vi "FTW-CodeGen-Initialize.vi"(5 "XRef":refnum<vi>) -> (4 "State Out":T1)   [LabVIEW 2015, in "FTW-dotNet-SQL-Insert.xnode"]
uses:
  FTW-dotNet-SQL-Insert.xnode
  FTW-CodeGen-State.ctl
panel:
  # "Inputs"
  # "Outputs"
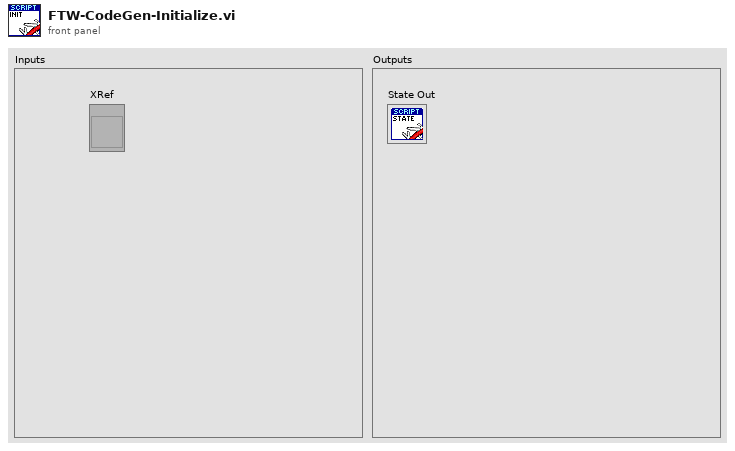
[diagram p1: front panel]
types:
  T1 = typedef "FTW-dotNet-SQL-Insert.xnode/FTW-CodeGen-State.ctl" = cluster{"Dummy":string}
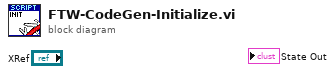
[diagram p0: block diagram]
diagram:
